vi "ApproveXCoord (SubVI).vi"(8 "Xhigh":dbl, 9 "Xlow":dbl, 11 "Go to X":dbl) -> (3 "Pass X?":bool)   [LabVIEW 2016]
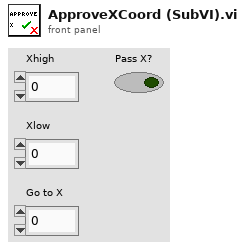
[diagram p1: front panel]
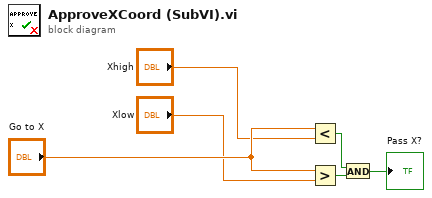
[diagram p0: block diagram]
diagram:
  n1 = Less?(x="Go to X", y="Xhigh") -> (x < y?=w3:bool)
  n2 = Greater?(x="Go to X", y="Xlow") -> (0:w2:bool)
  n3 = And(x=w3, y=w2) -> (x .and. y?=→"Pass X?":bool)
